vi "Truncate string to a given string length.vi"(5 "Max. Number of allowable characters":i32=30, 7 "Truncation Option":enum16{"Truncate the end"}(ring), 11 "String IN":string) -> (2 "Output String":string)   [LabVIEW 2022 SP3, in "Generic Utilities.lvclass"]
uses:
  Generic Utilities.lvclass
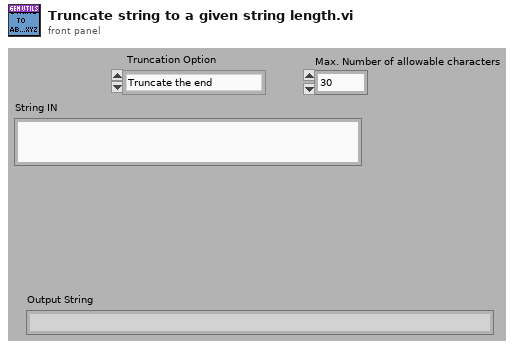
[diagram p1: front panel]
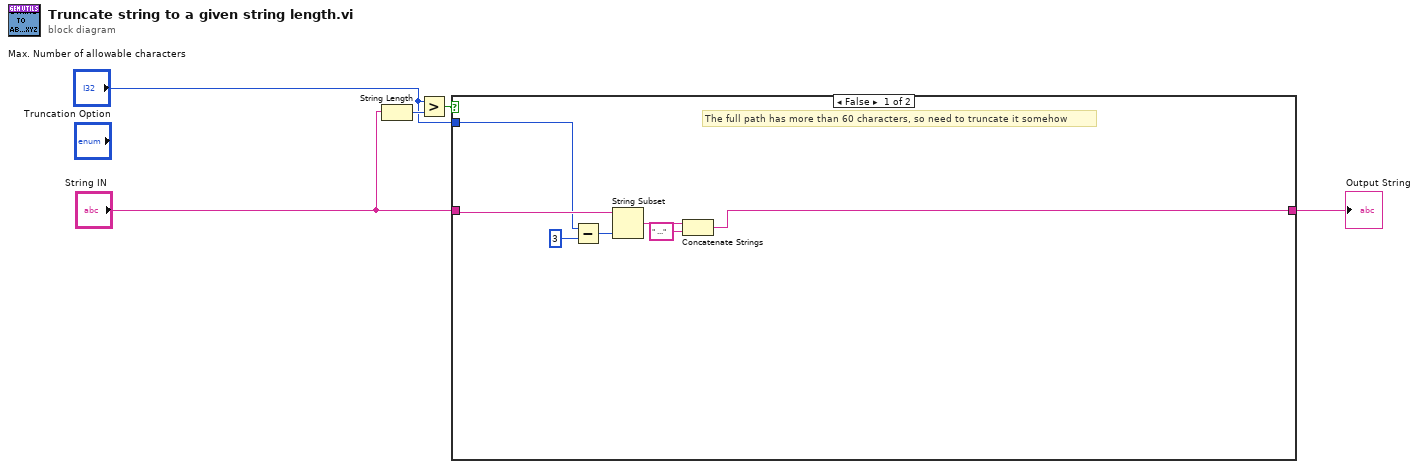
[diagram p0: block diagram]
diagram:
  n1 = String Length(string="String IN") -> (length=w3:i32)
  n2 = Greater?(x="Max. Number of allowable characters", y=w3) -> (0:w4:bool)
  n3 = case shown="False" w4 {
    tunnel: [w6 w13] -> w5
    tunnel: "String IN" -> [w12 w13]
    tunnel: "Max. Number of allowable characters" -> [w10 _]
    frame False {
      # "The full path has more than 60 characters, so need to truncate it somehow"
      n4 = Subtract(x=w10, y=3) -> (x-y=w11:i32)
      n5 = String Subset(string=w12, length (rest)=w11) -> (substring=w8:string)  [unwired: 1 in]
      n6 = Concatenate Strings(w8, " ..." ("string")) -> (w6:string)
    }
    frame True {
      # "The String has less than 30 characters, so do nothing"
    }
  }
  "Output String" <- w5
